vi "IDE copy.vi"() -> ()   [LabVIEW 2020]
uses:
  Subs/ColorText/Code.xctl
  Subs/Console XCtrl/Console_Xctrl.xctl
  Subs/Server XCtrl/Server.xctl
  Subs/SystemLink/SL_Subs/SL_XControl.xctl
  Subs/SystemLink/SL_Subs/SystemLink_Write_String.vi
panel:
  in  "SystemLink":string(xcontrol)="fred"
  in  "Clean":bool
  in  "PC Save":bool
  in  "PC path":path=path "/Users/CarterWS/Desktop/Senior Spring/CEEO/Project/temp.py"
  in  "Files":bool
  in  "Server":bool
  in  "Help":bool
  in  "Server":path(xcontrol)=path "/Users/CarterWS/Desktop/Senior Spring/CEEO/Summer2020/LabVIEWCode/Servers/Peter.vi"
  out "REPL":string(xcontrol)="NoneLinux ev3dev 4.14.117-ev3dev-2.3.5-ev3 #1 PREEMPT Sat Mar 7 12:54:39 CST 2020 armv5tejl\r\n             _____     _\r\n   _____   _|___ /  __| | _____   __\r\n  / _ \\ \\ / / |_ \\ / _` |/ _ \\ \\ / /\r\n |  __/\\ V / ___) | (_| |  __/\\ V /\r\n  \\___| \\_/ |____/ \\__,_|\\___| \\_/\r\n\r\nDebian stretch on LEGO MINDSTORMS EV3!\r\nLast login: Wed Jun  3 17:01:49 2020 from 192.168.7.106\r\r\n\r\n\r\nrobot@ev3dev:~$ \r\nrobot@ev3dev:~$ \r\nrobot@ev3dev:~$ brickrun -r --  pybricks-micropython\r\nPybricks MicroPython v1.11 on 2020-05-06; linux version\r\nUse Ctrl-D to exit, Ctrl-E for paste mode\r\n>>> import os\r\r\n>>> "
  in  "Clear":bool
  in  "Save":bool
  in  "Stop":bool
  in  "Run":bool=TRUE
  in  "Name":string="temp.py"
  in  "Code":string(xcontrol)="#!/usr/bin/env pybricks-micropython\n\nfrom pybricks import ev3brick as brick\nfrom pybricks.ev3devices import (Motor, TouchSensor, \n    ColorSensor,InfraredSensor, UltrasonicSensor, GyroSensor)\nfrom pybricks.parameters import (Port, Stop, Direction, Button, Color,\n    SoundFile, ImageFile, Align)\nfrom pybricks.tools import print, wait, StopWatch\nfrom pybricks.robotics import DriveBase\nimport time"
  # "¨Processor"
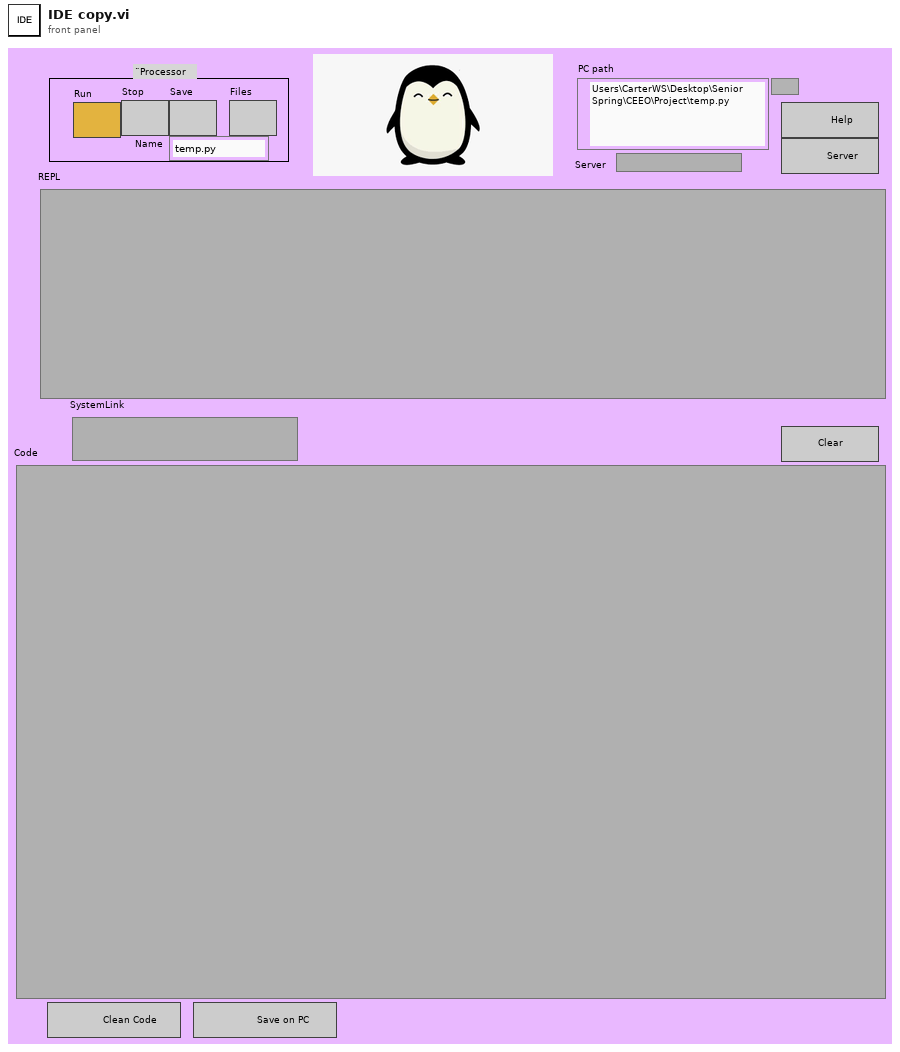
[diagram p1: front panel]
types:
  T1 = cluster{"Quote":u32, "Comment":u32, "Python":u32, "Text":u32, "Triple Quote":u32, "function":u32, "Line numbers":u32, "REPL Err":u32, "REPL Text":u32, "Text Bkgd":u32, "REPL Bkgd":u32}
  T2 = enum8{"Enabled", "Disabled", "Disabled and Grayed Out"}
  T3 = typedef "eventvkey.ctl" = enum16{"ASCII", "Enter", "Return", "Shift", "Ctrl", "Alt", "Cmd", "Opt", "Caps", "NumLock", "Clear", "Break", "Up", "Down", "Left", "Right", "Insert", "Delete", "Home", "End", "PageUp", "PageDown", "Escape", "Help", "Pause", "ScrollLock", "F1", "F2", "F3", "F4", "F5", "F6", "F7", "F8", "F9", "F10", "F11", "F12", "F13", "F14", "F15", "F16", "F17", "F18", "F19", "F20", "F21", "F22", "F23", "F24", "Play", "VolumeUp", "VolumeDown", "Mute", "Two Byte Char"}
  T4 = cluster{"Shift":bool, "Ctrl":bool, "Alt":bool, "Cmd":bool, "Opt":bool}
  T5 = cluster{"Char":i16, "VKey":T3, "PlatMods":cluster{"Shift":bool, "Ctrl":bool, "Alt":bool, "Cmd":bool, "Opt":bool}}
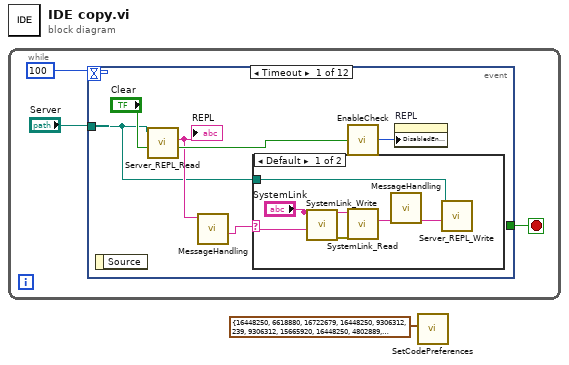
[diagram p0: block diagram]
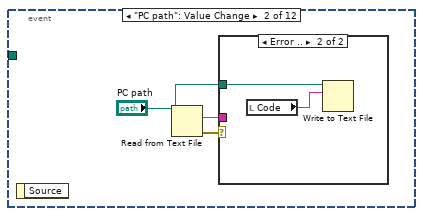
[diagram p3: hidden frame]
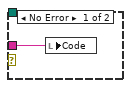
[diagram p4: hidden frame]
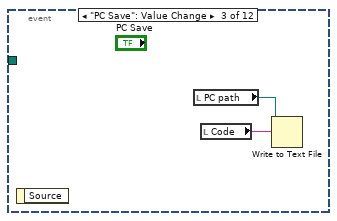
[diagram p5: hidden frame]
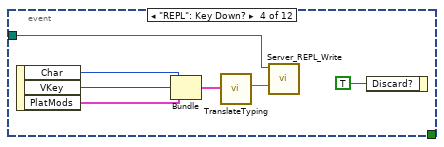
[diagram p6: hidden frame]
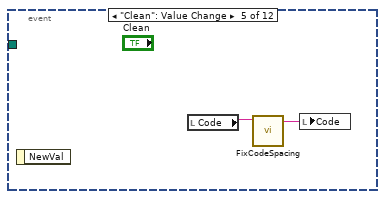
[diagram p7: hidden frame]
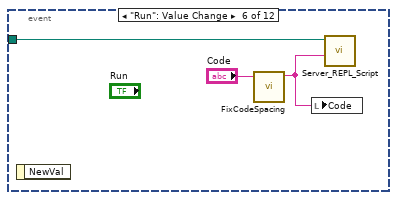
[diagram p8: hidden frame]
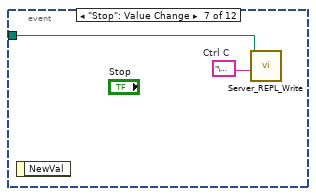
[diagram p9: hidden frame]
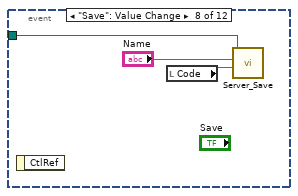
[diagram p10: hidden frame]
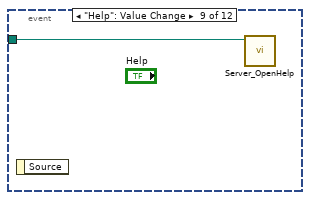
[diagram p11: hidden frame]
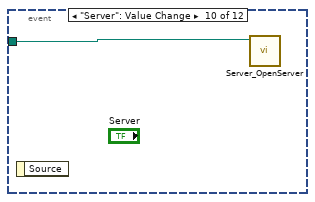
[diagram p12: hidden frame]
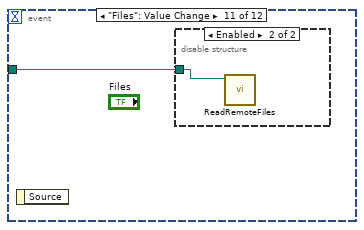
[diagram p13: hidden frame]
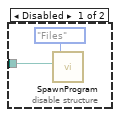
[diagram p14: hidden frame]
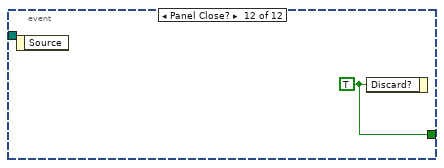
[diagram p15: hidden frame]
diagram:
  n1 = while {
    stop <- w3 stop-if-true
    n2 = event shown="[0] Timeout" {
      selector: _ -> [_ _ _ _ _ _ _ _ _ _ _ _]
      dyn-events: _ -> [_ _ _ _ _ _ _ _ _ _ _ _]
      timeout: 100 -> [_ _ _ _ _ _ _ _ _ _ _ _]
      tunnel: [_ _ _ _ _ _ _ _ _ _ _ w48] -> w3
      tunnel: "Server" -> [w5 _ _ w25 _ w35 w37 w39 w42 w43 w44 _]
      event Timeout {
        n3 = event-data() -> ()  [unwired: 1 in, 1 out]
        n4 = call "Server_REPL_Read.vi"("Clear"="Clear", "Server"=w5) -> ("Running?"=w9:bool, "REPL"=w7:string)  [unwired: 7 in, 1 out]
        "REPL" <- w7
        n5 = call "MessageHandling.vi"("REPL"=w7) -> ("New Message"=w6:string)  [unwired: 7 in, 3 out]
        n6 = case shown="Default" w6 {
          selector: w6 -> [w12 _]
          tunnel: w5 -> [w14 _]
          frame Default {
            n7 = call-poly "SystemLink_Write.vi"("String"=w12, "SL_XControl"="SystemLink") -> ("error out"=w16:errorcluster)  [unwired: 9 in]
            n8 = call "SystemLink_Read.vi"("error in"=w16, "SystemLink Tag"="SystemLink") -> ("value"=w11:string)  [unwired: 6 in, 3 out]
            n9 = call "MessageHandling.vi"("Reply"=w11) -> ("New Reply"=w13:string)  [unwired: 7 in, 3 out]
            n10 = call "Server_REPL_Write.vi"("Code"=w13, "Server"=w14) -> ()  [unwired: 9 in, 1 out]
          }
          frame "" {
          }
        }
        n11 = call "EnableCheck.vi"("Enable?"=w9) -> ("Enum"=w10:T2)
        n12 = property on="REPL" class="Console_Xctrl (strict)"("DisabledEnum"=w10) -> ()  [unwired: 2 in, 2 out]
      }
      event "PC path": Value Change {
        n13 = event-data() -> ()  [unwired: 1 in, 1 out]
        n14 = Read from Text File(file (use dialog)="PC path") -> (text=w18:string, error out=w19:errorcluster)  [unwired: 3 in, 2 out]
        n15 = case shown="Error .." w19 {
          tunnel: w18 -> [w20 _]
          tunnel: "PC path" -> [_ w22]
          frame No Error {
            n16 = local write "Code"(w20) -> ()
          }
          frame Error {
            n17 = local read "Code"() -> (w21:string)
            n18 = Write to Text File(file (use dialog)=w22, text=w21) -> ()  [unwired: 2 in, 3 out]
          }
        }
      }
      event "PC Save": Value Change {
        n19 = event-data() -> ()  [unwired: 1 in, 1 out]
        n20 = local read "PC path"() -> (w24:path)
        n21 = local read "Code"() -> (w23:string)
        n22 = Write to Text File(file (use dialog)=w24, text=w23) -> ()  [unwired: 2 in, 3 out]
      }
      event "REPL": Key Down? {
        n23 = event-data() -> ("Char"=w30:i16, "VKey"=w29:T3, "PlatMods"=w27:T4)  [unwired: 1 in]
        n24 = Bundle("Char"=w30, "VKey"=w29, "PlatMods"=w27) -> (w31:T5)  [unwired: 1 in]
        n25 = call "TranslateTyping.vi"("Cluster"=w31) -> ("key"=w26:string)  [unwired: 10 in]
        n26 = call "Server_REPL_Write.vi"("Code"=w26, "Server"=w25) -> ()  [unwired: 9 in, 1 out]
        n27 = event-data("Discard?"=TRUE) -> ()  [unwired: 1 in, 1 out]
      }
      event "Clean": Value Change {
        n28 = event-data() -> ()  [unwired: 1 in, 1 out]
        n29 = local read "Code"() -> (w32:string)
        n30 = call "FixCodeSpacing.vi"("Code"=w32) -> ("Cleaned"=w33:string)  [unwired: 10 in]
        n31 = local write "Code"(w33) -> ()
      }
      event "Run": Value Change {
        n32 = event-data() -> ()  [unwired: 1 in, 1 out]
        n33 = call "FixCodeSpacing.vi"("Code"="Code") -> ("Cleaned"=w34:string)  [unwired: 10 in]
        n34 = local write "Code"(w34) -> ()
        n35 = call "Server_REPL_Script.vi"("Code"=w34, "Server"=w35) -> ()  [unwired: 9 in, 1 out]
      }
      event "Stop": Value Change {
        w38 = "\u0003"  # Ctrl C
        n36 = event-data() -> ()  [unwired: 1 in, 1 out]
        n37 = call "Server_REPL_Write.vi"("Code"=w38, "Server"=w37) -> ()  [unwired: 9 in, 1 out]
      }
      event "Save": Value Change {
        n38 = event-data() -> ()  [unwired: 1 in, 1 out]
        n39 = local read "Code"() -> (w41:string)
        n40 = call "Server_Save.vi"("Code"=w41, "Name"="Name", "Server"=w39) -> ()  [unwired: 8 in, 1 out]
      }
      event "Help": Value Change {
        n41 = event-data() -> ()  [unwired: 1 in, 1 out]
        n42 = call "Server_OpenHelp.vi"("Server"=w42) -> ()  [unwired: 10 in, 1 out]
      }
      event "Server": Value Change {
        n43 = event-data() -> ()  [unwired: 1 in, 1 out]
        n44 = call "Server_OpenServer.vi"("Server"=w43) -> ()  [unwired: 10 in, 1 out]
      }
      event "Files": Value Change {
        n45 = event-data() -> ()  [unwired: 1 in, 1 out]
        n46 = disable-structure shown="Enabled" {
          disable-tunnel: w44 -> [w45 w47]
          frame Disabled {
            n47 = call "SpawnProgram.vi"("Server"=w45, "Dialog"=enum16{"Help", "Files"}."Files") -> ()  [unwired: 10 in]
          }
          frame Enabled {
            n48 = call "ReadRemoteFiles.vi"("Server"=w47) -> ()  [unwired: 11 in]
          }
        }
      }
      event Panel Close? {
        w48 = TRUE ("Discard?")
        n49 = event-data() -> ()  [unwired: 1 in, 1 out]
        n50 = event-data("Discard?"=w48) -> ()  [unwired: 1 in, 1 out]
      }
    }
  }
  n51 = call "SetCodePreferences.vi"("Color choices"=T1 {"Quote"=16448250, "Comment"=6618880, "Python"=16722679, "Text"=16448250, "Triple Quote"=9306312, "function"=239, "Line numbers"=9306312, "REPL Err"=15665920, "REPL Text"=16448250, "Text Bkgd"=4802889, "REPL Bkgd"=4802889}) -> ()  [unwired: 11 in]
